vi "Index_Logic.vi"(4 "Intake Pressed":bool, 5 "X":bool, 6 "B":bool, 7 "Right Trigger":dbl, 8 "Y":bool, 9 "A":bool, 11 "Elevate Pressed":bool) -> ()   [LabVIEW 2020]
uses:
  <vilib>/Rock Robotics/WPI/ThirdParty/Phoenix-LabVIEW/Motor Controller/Controls/CTRE_Phoenix_MotorControl_ControlMode.ctl
  <vilib>/Rock Robotics/Network Tables/NT Read String.vi
  <vilib>/Rock Robotics/Network Tables/NT Write Boolean.vi
  <vilib>/Rock Robotics/Network Tables/NT Write Number.vi
panel:
  in  "Intake want":dbl=0.8
  in  "Elevate want":dbl=-0.35
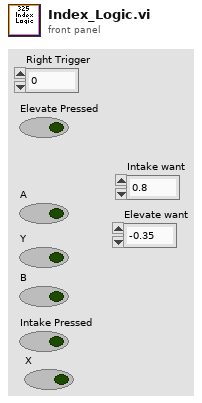
[diagram p1: front panel]
types:
  T1 = typedef "CTRE_Phoenix_MotorControl_ControlMode.ctl" = u16
  T2 = typedef "WPI_MotorControlDeviceRef.ctl" = cluster{"DeviceStatus":errorcluster, "Type":T3, "PWM":cluster{"PWM Channel":T4, "DeadBand":T5}, "CAN":cluster{"Device Number":u8, "SetOutput VI Ref":variant, "GetOutput VI Ref":variant, "Enable VI Ref":variant, "Disable VI Ref":variant, "Data":variant}, "Invert":bool, "DIO PWM":cluster{"PWM \"Enable\" Channel":T4, "DIOChannel":T6, "PWM Rate":dbl}}
  T3 = typedef "WPI_MotorControlType.ctl" = enum16{"PWM", "CAN", "DIO PWM"}
  T4 = typedef "FPGA_DIOPWMChannel.ctl" = enum8{"PWM 0", "PWM 1", "PWM 2", "PWM 3", "PWM 4", "PWM 5", "PWM 6", "PWM 7", "PWM 8", "PWM 9", "PWM MXP 0", "PWM MXP 1", "PWM MXP 2", "PWM MXP 3", "PWM MXP 4", "PWM MXP 5", "PWM MXP 6", "PWM MXP 7", "PWM MXP 8", "PWM MXP 9", "Invalid"}
  T5 = typedef "WPI_PWMDeadband.ctl" = cluster{"Name":string, "maxPositivePwm":i32, "minPositivePwm":i32, "centerPwm":i32, "maxNegativePwm":i32, "minNegativePwm":i32, "angularRange":u16}
  T6 = typedef "FPGA_DIOChannel.ctl" = enum8{"DIO 0", "DIO 1", "DIO 2", "DIO 3", "DIO 4", "DIO 5", "DIO 6", "DIO 7", "DIO 8", "DIO 9", "DIO MXP 0", "DIO MXP 1", "DIO MXP 2", "DIO MXP 3", "DIO MXP 4", "DIO MXP 5", "DIO MXP 6", "DIO MXP 7", "DIO MXP 8", "DIO MXP 9", "DIO MXP 10", "DIO MXP 11", "DIO MXP 12", "DIO MXP 13", "DIO MXP 14", "DIO MXP 15", "SPI Port CS1", "SPI Port CS2", "SPI Port CS3", "SPI Port MISO", "SPI Port MOSI", "Invalid"}
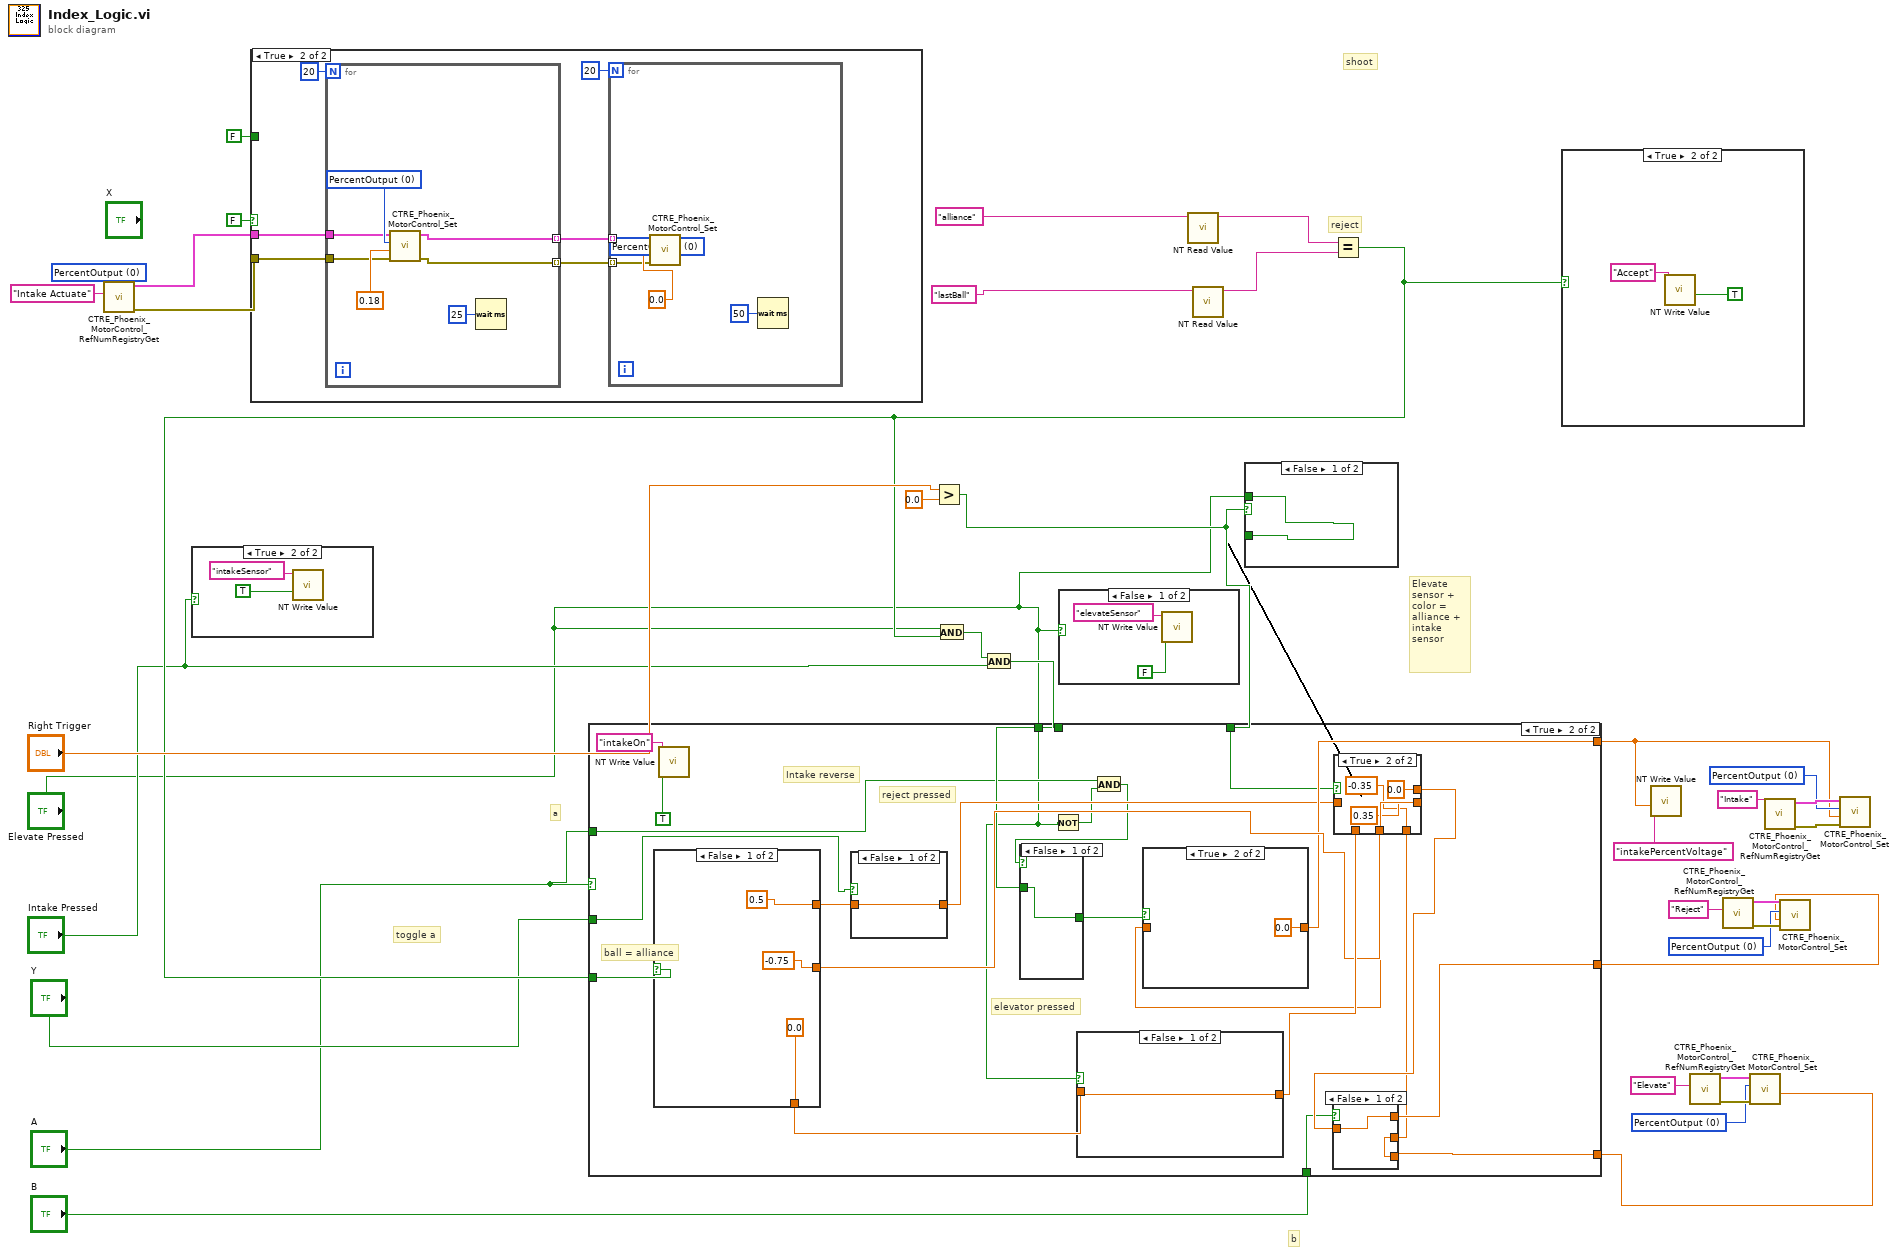
[diagram p0: block diagram]
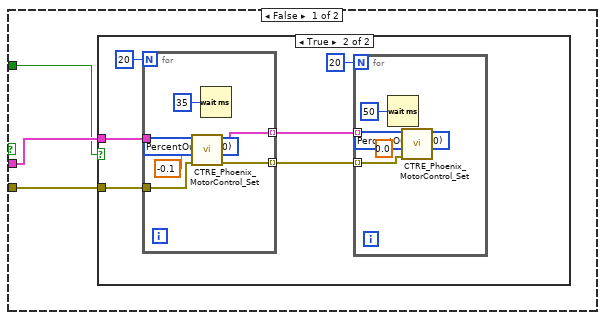
[diagram p2: hidden frame]
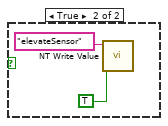
[diagram p4: hidden frame]
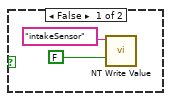
[diagram p5: hidden frame]
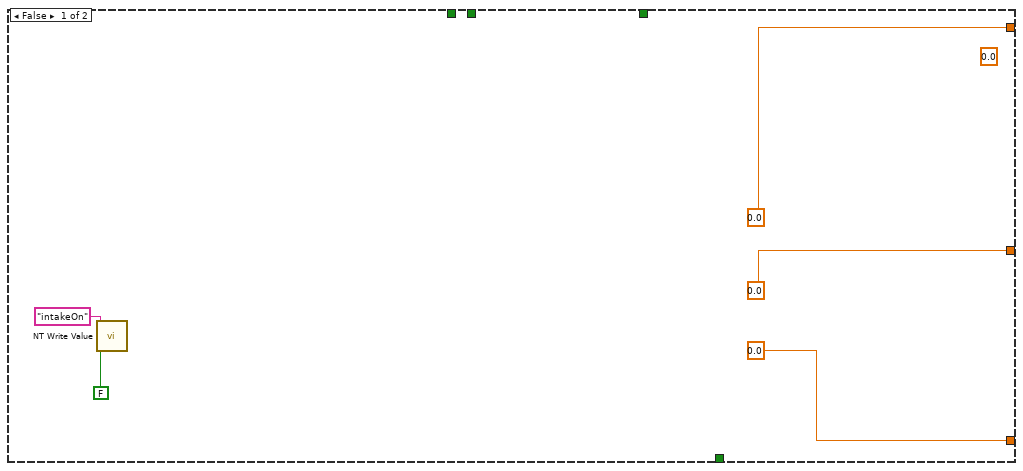
[diagram p6: hidden frame]
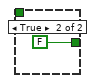
[diagram p7: hidden frame]
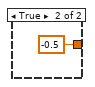
[diagram p8: hidden frame]
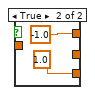
[diagram p9: hidden frame]
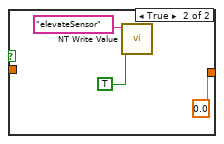
[diagram p12: hidden frame]
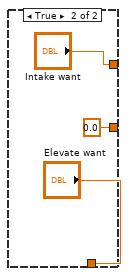
[diagram p13: hidden frame]
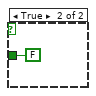
[diagram p14: hidden frame]
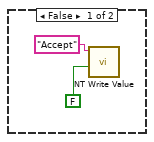
[diagram p15: hidden frame]
diagram:
  (unwired) T1 0 items=["PercentOutput"=0, "Position"=1, "Velocity"=2, "Current"=3, "Follower"=5, "MotionProfile"=6, "MotionMagic"=7, "MotionProfileArc"=10, "Disabled"=15] ("Control Mode")
  w25 = T1 0 items=["PercentOutput"=0, "Position"=1, "Velocity"=2, "Current"=3, "Follower"=5, "MotionProfile"=6, "MotionMagic"=7, "MotionProfileArc"=10, "Disabled"=15] ("Control Mode")
  w26 = T1 0 items=["PercentOutput"=0, "Position"=1, "Velocity"=2, "Current"=3, "Follower"=5, "MotionProfile"=6, "MotionMagic"=7, "MotionProfileArc"=10, "Disabled"=15] ("Control Mode")
  w27 = T1 0 items=["PercentOutput"=0, "Position"=1, "Velocity"=2, "Current"=3, "Follower"=5, "MotionProfile"=6, "MotionMagic"=7, "MotionProfileArc"=10, "Disabled"=15] ("Control Mode")
  # "toggle a"
  # "Elevate sensor + color = alliance + intake sensor"
  # "b"
  # "a"
  # "shoot"
  # "reject"
  n1 = call <vilib>:"CTRE_Phoenix_MotorControl_RefNumRegistryGet.vi"("refnum name"="Intake Actuate") -> ("error out"=w5:errorcluster, "PhoenixMotorControlDevRef"=w6:T2)  [unwired: 9 in]
  n2 = case shown="True" "Intake Pressed" {
    frame False {
      n3 = call-poly <vilib>:"NT Write Value.vi"("Boolean"=FALSE, "Name"="intakeSensor") -> ()  [unwired: 9 in, 1 out]
    }
    frame True {
      n4 = call-poly <vilib>:"NT Write Value.vi"("Boolean"=TRUE, "Name"="intakeSensor") -> ()  [unwired: 9 in, 1 out]
    }
  }
  n5 = case shown="True" FALSE {
    tunnel: w6 -> [w43 w66]
    tunnel: w5 -> [w42 w63]
    tunnel: FALSE ("X") -> [w41 _]
    frame False {
      n6 = case shown="True" w41 {
        tunnel: w43 -> [_ w49]
        tunnel: w42 -> [_ w48]
        frame False {
        }
        frame True {
          n7 = for {
            N: 20 -> [_]
            tunnel: w49 -> [w61]
            tunnel: w48 -> [w60]
            tunnel: [w59] -> w47 mode=indexing
            tunnel: [w58] -> w46 mode=indexing
            w56 = T1 0 items=["PercentOutput"=0, "Position"=1, "Velocity"=2, "Current"=3, "Follower"=5, "MotionProfile"=6, "MotionMagic"=7, "MotionProfileArc"=10, "Disabled"=15] ("Control Mode")
            n8 = call <vilib>:"CTRE_Phoenix_MotorControl_Set.vi"("error in (no error)"=w60, "Output"=-0.1, "Control Mode"=w56, "PhoenixMotorControlDevRef"=w61) -> ("error out"=w58:errorcluster, "PhoenixMotorControlDevRef"=w59:T2)  [unwired: 6 in]
            n9 = Wait (ms)(milliseconds to wait=u32 35) -> ()  [unwired: 1 out]
          }
          n10 = for {
            N: 20 -> [_]
            tunnel: w47 -> [w54] mode=indexing
            tunnel: w46 -> [w53] mode=indexing
            w51 = T1 0 items=["PercentOutput"=0, "Position"=1, "Velocity"=2, "Current"=3, "Follower"=5, "MotionProfile"=6, "MotionMagic"=7, "MotionProfileArc"=10, "Disabled"=15] ("Control Mode")
            n11 = Wait (ms)(milliseconds to wait=u32 50) -> ()  [unwired: 1 out]
            n12 = call <vilib>:"CTRE_Phoenix_MotorControl_Set.vi"("error in (no error)"=w53, "Output"=0.0, "Control Mode"=w51, "PhoenixMotorControlDevRef"=w54) -> ()  [unwired: 6 in, 2 out]
          }
        }
      }
    }
    frame True {
      n13 = for {
        N: 20 -> [_]
        tunnel: w66 -> [w76]
        tunnel: [w75] -> w65 mode=indexing
        tunnel: [w74] -> w64 mode=indexing
        tunnel: w63 -> [w73]
        w77 = T1 0 items=["PercentOutput"=0, "Position"=1, "Velocity"=2, "Current"=3, "Follower"=5, "MotionProfile"=6, "MotionMagic"=7, "MotionProfileArc"=10, "Disabled"=15] ("Control Mode")
        n14 = call <vilib>:"CTRE_Phoenix_MotorControl_Set.vi"("error in (no error)"=w73, "Output"=0.18, "Control Mode"=w77, "PhoenixMotorControlDevRef"=w76) -> ("error out"=w74:errorcluster, "PhoenixMotorControlDevRef"=w75:T2)  [unwired: 6 in]
        n15 = Wait (ms)(milliseconds to wait=u32 25) -> ()  [unwired: 1 out]
      }
      n16 = for {
        N: 20 -> [_]
        tunnel: w65 -> [w69] mode=indexing
        tunnel: w64 -> [w68] mode=indexing
        w70 = T1 0 items=["PercentOutput"=0, "Position"=1, "Velocity"=2, "Current"=3, "Follower"=5, "MotionProfile"=6, "MotionMagic"=7, "MotionProfileArc"=10, "Disabled"=15] ("Control Mode")
        n17 = call <vilib>:"CTRE_Phoenix_MotorControl_Set.vi"("error in (no error)"=w68, "Output"=0.0, "Control Mode"=w70, "PhoenixMotorControlDevRef"=w69) -> ()  [unwired: 6 in, 2 out]
        n18 = Wait (ms)(milliseconds to wait=u32 50) -> ()  [unwired: 1 out]
      }
    }
  }
  n19 = Greater?(x="Right Trigger", y=0.0) -> (0:w15:bool)
  n20 = case shown="False" "Elevate Pressed" {
    frame False {
      n21 = call-poly <vilib>:"NT Write Value.vi"("Boolean"=FALSE, "Name"="elevateSensor") -> ()  [unwired: 9 in, 1 out]
    }
    frame True {
      n22 = call-poly <vilib>:"NT Write Value.vi"("Boolean"=TRUE, "Name"="elevateSensor") -> ()  [unwired: 9 in, 1 out]
    }
  }
  n23 = call-poly <vilib>:"NT Read Value.vi"("Name"="alliance") -> ("String"=w24:string)  [unwired: 9 in, 1 out]
  n24 = call-poly <vilib>:"NT Read Value.vi"("Name"="lastBall") -> ("String"=w21:string)  [unwired: 9 in, 1 out]
  n25 = case shown="False" w15 {
    tunnel: "Elevate Pressed" -> [w84 _]
    tunnel: [w84 FALSE ("Switch Pressed")] -> _
    frame False {
    }
    frame True {
    }
  }
  n26 = Equal?(x=w24, y=w21) -> (x = y?=w12:bool)
  n27 = And(x="Elevate Pressed", y=w12) -> (x .and. y?=w18:bool)
  n28 = And(x=w18, y="Intake Pressed") -> (x .and. y?=w17:bool)
  n29 = case shown="True" "A" {
    tunnel: w12 -> [_ w113]
    tunnel: [0.0 ("Intake want") w100] -> w8
    tunnel: [0.0 ("Elevate 1") w107] -> w20
    tunnel: "Elevate Pressed" -> [_ w93]
    tunnel: [0.0 ("Reject no want") w109] -> w19
    tunnel: w17 -> [_ w96]
    tunnel: w15 -> [_ w97]
    tunnel: "B" -> [_ w108]
    tunnel: "Y" -> [_ w106]
    tunnel: "A" -> [_ w94]
    frame False {
      (unwired) 0.0 ("Output")
      n30 = call-poly <vilib>:"NT Write Value.vi"("Boolean"=FALSE, "Name"="intakeOn") -> ()  [unwired: 9 in, 1 out]
    }
    frame True {
      # "Intake reverse"
      # "reject pressed"
      # "elevator pressed"
      # "ball = alliance"
      n31 = case shown="False" w113 {
        tunnel: [0.0 ("Elevate want") "Elevate want"] -> w112
        tunnel: [0.5 ("Intake 1") "Intake want"] -> w105
        tunnel: [-0.75 ("Reject no want") 0.0 ("Reject no want")] -> w102
        frame False {
        }
        frame True {
        }
      }
      n32 = call-poly <vilib>:"NT Write Value.vi"("Boolean"=TRUE, "Name"="intakeOn") -> ()  [unwired: 9 in, 1 out]
      n33 = case shown="False" w106 {
        tunnel: [w116 -0.5 ("Intake want")] -> w98
        tunnel: w105 -> [w116 _]
        frame False {
        }
        frame True {
        }
      }
      n34 = Not(x=w93) -> (.not. x?=w95:bool)
      n35 = case shown="False" w93 {
        tunnel: [w130 0.0 ("Elevate 1")] -> w111
        tunnel: w112 -> [w130 _]
        frame False {
        }
        frame True {
          n36 = call-poly <vilib>:"NT Write Value.vi"("Boolean"=TRUE, "Name"="elevateSensor") -> ()  [unwired: 9 in, 1 out]
        }
      }
      n37 = And(x=w94, y=w95) -> (x .and. y?=w92:bool)
      n38 = case shown="False" w92 {
        tunnel: w96 -> [w114 _]
        tunnel: [w114 FALSE ("Boolean")] -> w91
        frame False {
        }
        frame True {
        }
      }
      n39 = case shown="True" w97 {
        tunnel: w98 -> [w124 _]
        tunnel: [w124 0.35 ("Intake want")] -> w99
        tunnel: w111 -> [w123 _]
        tunnel: [w123 -0.35 ("Elevate 1")] -> w101
        tunnel: w102 -> [w122 _]
        tunnel: [w122 0.0 ("Reject no want")] -> w110
        frame False {
        }
        frame True {
        }
      }
      n40 = case shown="True" w91 {
        tunnel: w99 -> [w128 _]
        tunnel: [w128 0.0 ("Intake want")] -> w100
        frame False {
        }
        frame True {
        }
      }
      n41 = case shown="False" w108 {
        tunnel: w110 -> [w119 _]
        tunnel: [w119 -1.0 ("Reject no want")] -> w109
        tunnel: [w118 1.0 ("Elevate 1")] -> w107
        tunnel: w101 -> [w118 _]
        frame False {
        }
        frame True {
        }
      }
    }
  }
  n42 = case shown="True" w12 {
    frame False {
      n43 = call-poly <vilib>:"NT Write Value.vi"("Boolean"=FALSE, "Name"="Accept") -> ()  [unwired: 9 in, 1 out]
    }
    frame True {
      n44 = call-poly <vilib>:"NT Write Value.vi"("Boolean"=TRUE, "Name"="Accept") -> ()  [unwired: 9 in, 1 out]
    }
  }
  n45 = call-poly <vilib>:"NT Write Value.vi"("Numeric"=w8, "Name"="intakePercentVoltage") -> ()  [unwired: 9 in, 1 out]
  n46 = call <vilib>:"CTRE_Phoenix_MotorControl_RefNumRegistryGet.vi"("refnum name"="Elevate") -> ("error out"=w32:errorcluster, "PhoenixMotorControlDevRef"=w31:T2)  [unwired: 9 in]
  n47 = call <vilib>:"CTRE_Phoenix_MotorControl_RefNumRegistryGet.vi"("refnum name"="Reject") -> ("error out"=w34:errorcluster, "PhoenixMotorControlDevRef"=w33:T2)  [unwired: 9 in]
  n48 = call <vilib>:"CTRE_Phoenix_MotorControl_Set.vi"("error in (no error)"=w32, "Output"=w20, "Control Mode"=w27, "PhoenixMotorControlDevRef"=w31) -> ()  [unwired: 6 in, 2 out]
  n49 = call <vilib>:"CTRE_Phoenix_MotorControl_RefNumRegistryGet.vi"("refnum name"="Intake") -> ("error out"=w36:errorcluster, "PhoenixMotorControlDevRef"=w35:T2)  [unwired: 9 in]
  n50 = call <vilib>:"CTRE_Phoenix_MotorControl_Set.vi"("error in (no error)"=w34, "Output"=w19, "Control Mode"=w25, "PhoenixMotorControlDevRef"=w33) -> ()  [unwired: 6 in, 2 out]
  n51 = call <vilib>:"CTRE_Phoenix_MotorControl_Set.vi"("error in (no error)"=w36, "Output"=w8, "Control Mode"=w26, "PhoenixMotorControlDevRef"=w35) -> ()  [unwired: 6 in, 2 out]
